vi "estadoToneBurst.vi"(8 "error in (no error)":errorcluster, 10 "Tm":i32=60, 11 "N":i32=1) -> (0 "error out":errorcluster, 2 "Terminar":bool)   [LabVIEW 2019, in "Prueba08.lvclass"]
uses:
  Prueba08.lvclass
panel:
  out "Tm":i32=60
  out "seg":i32=60
  in  "terminar":bool
  out "N_actual":i32
  out "N":i32=1
  out "estado":string
  # "Repeticiones que debe hacer"
  # "Repetición actual"
  # "Tiempo de la prueba (seg)"
  # "Tiempo transcurrido (seg)"
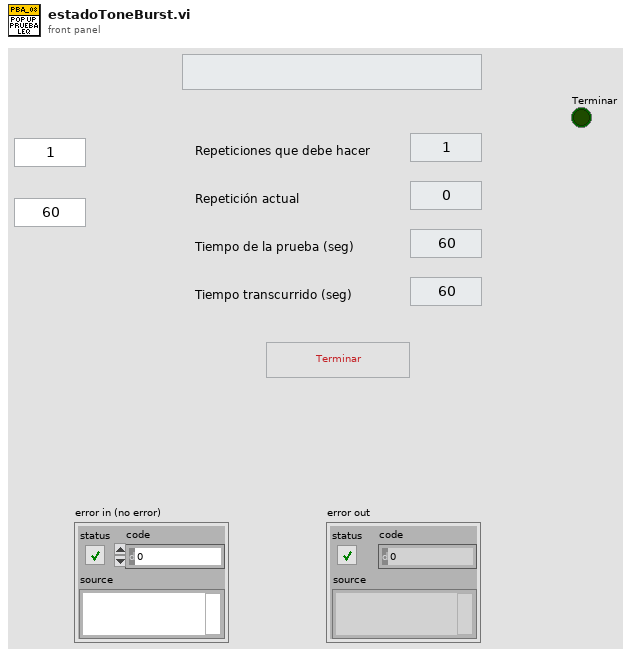
[diagram p1: front panel]
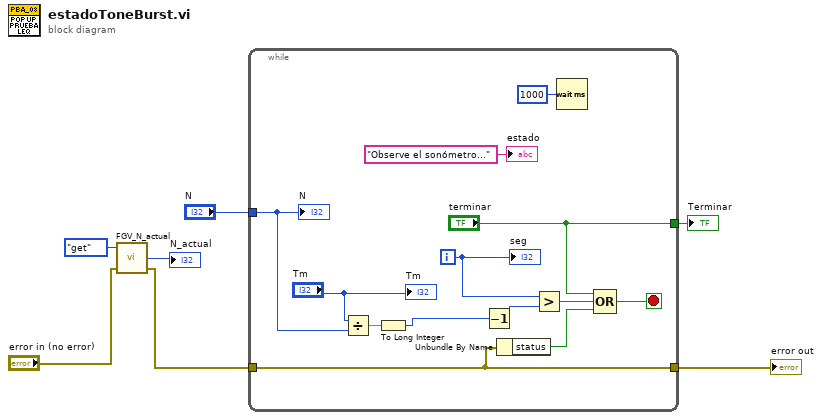
[diagram p0: block diagram]
diagram:
  n1 = call "FGV_N_actual.vi"("error in (no error)"="error in (no error)", "action"=enum16{"increment", "set_start", "get"}."get") -> ("error out"=w3:errorcluster, "N_actual out"=→"N_actual":i32)  [unwired: 2 in]
  n2 = while {
    tunnel: "N" -> [w13]
    tunnel: w3 -> [w9]
    tunnel: [w9] -> w2
    tunnel: ["terminar"] -> w1
    i -> [w19]
    stop <- w16 stop-if-true
    n3 = Divide(x="Tm", y=w13) -> (x/y=w12:dbl)
    n4 = To Long Integer(number=w12) -> (32bit integer=w11:i32)
    n5 = Decrement(x=w11) -> (x-1=w15:i32)
    n6 = Unbundle By Name(w9) -> ("status"=w10:bool)
    n7 = Greater?(x=w19, y=w15) -> (0:w17:bool)
    n8 = Wait (ms)(milliseconds to wait=u32 1000) -> ()  [unwired: 1 out]
    n9 = Compound Arithmetic op=OR("terminar", w17, w10) -> (w16:bool)
    "estado" <- "Observe el sonómetro..." ("estado")
    "seg" <- w19
    "N" <- w13
    "Tm" <- "Tm"
  }
  "error out" <- w2
  "Terminar" <- w1
